vi "Configure Event Search (Serial Bus - A429).vi"(5 "SSM Pattern (00)":string="00", 6 "SDI Pattern (00)":string="00", 7 "Data Pattern (0000000000000000000)":string="0000000000000000000", 8 "error in (no error)":errorcluster, 9 "Label Value (0)":i32, 10 "Search Operation (0: Label)":i32(ring) items=["Label", "Label Bits", "Parity Error", "Word Error", "Gap Error", "Word or Gap Errors", "All Errors"], 11 "VISA resource name":refnum<visa-resource-name>) -> (0 "error out":errorcluster, 3 "VISA resource name out":refnum<visa-resource-name>)   [LabVIEW 2010, in "Agilent 2000 3000 X-Series.lvlib"]
doc: "Configures the event search of ARINC 429 bus."
uses:
  <instrlib>/Agilent 2000 3000 X-Series/Agilent 2000 3000 X-Series.lvlib
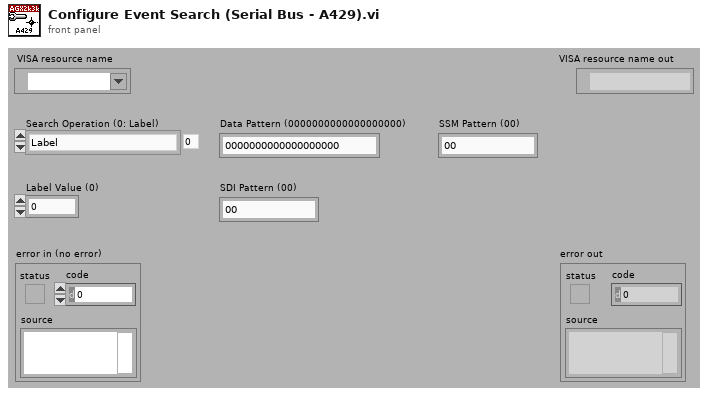
[diagram p1: front panel]
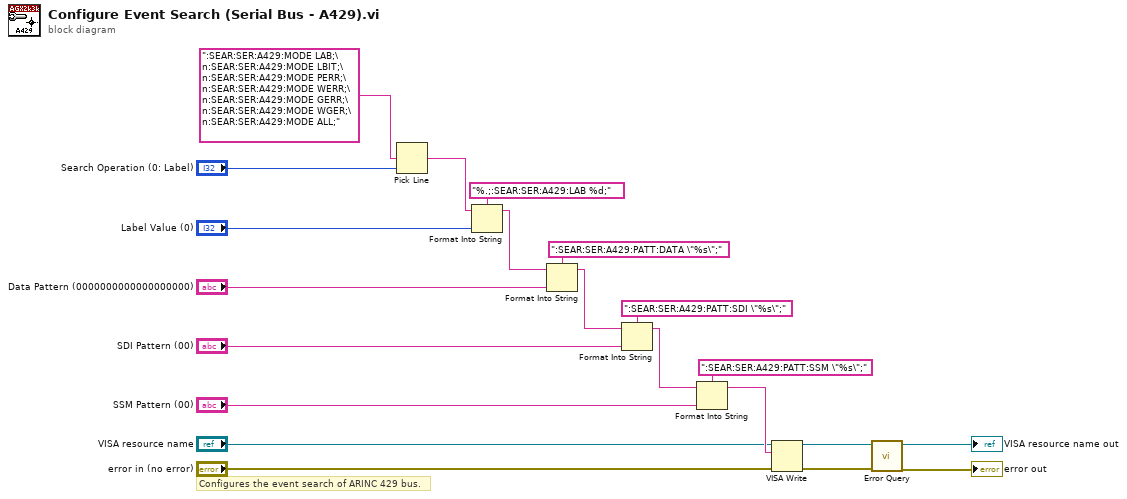
[diagram p0: block diagram]
diagram:
  # "Configures the event search of ARINC 429 bus."
  n1 = Pick Line(multi-line string=":SEAR:SER:A429:MODE LAB;\n:SEAR:SER:A429:MODE LBIT;\n:SEAR:SER:A429:MODE PERR;\n:SEAR:SER:A429:MODE WERR;\n:SEAR:SER:A429:MODE GERR;\n:SEAR:SER:A429:MODE WGER;\n:SEAR:SER:A429:MODE ALL;", line index="Search Operation (0: Label)") -> (output string=w19:string)  [unwired: 1 out]
  n2 = Format Into String(format string="%.;:SEAR:SER:A429:LAB %d;", initial string=w19, "Label Value (0)") -> (resulting string=w16:string)  [unwired: 1 in, 1 out]
  n3 = Format Into String(format string=":SEAR:SER:A429:PATT:DATA \"%s\";", initial string=w16, "Data Pattern (0000000000000000000)") -> (resulting string=w13:string)  [unwired: 1 in, 1 out]
  n4 = Format Into String(format string=":SEAR:SER:A429:PATT:SDI \"%s\";", initial string=w13, "SDI Pattern (00)") -> (resulting string=w10:string)  [unwired: 1 in, 1 out]
  n5 = Format Into String(format string=":SEAR:SER:A429:PATT:SSM \"%s\";", initial string=w10, "SSM Pattern (00)") -> (resulting string=w7:string)  [unwired: 1 in, 1 out]
  n6 = VISA Write(VISA resource name="VISA resource name", write buffer=w7, error in (no error)="error in (no error)") -> (VISA resource name out=w4:refnum<visa-resource-name>, error out=w3:errorcluster)  [unwired: 1 out]
  n7 = call <instrlib>:"Error Query.vi"("error in (no error)"=w3, "VISA resource name"=w4) -> ("error out"=→"error out":errorcluster, "VISA resource name out"=→"VISA resource name out":refnum<visa-resource-name>)  [unwired: 8 out]
